vi "Create Landscape.vi"(9 "offset":i32, 10 "Column":i32, 11 "Row":i32) -> ()   [LabVIEW 2016, in "Defenders.lvclass"]
uses:
  Defenders.lvclass
  Terrain.ctl
  Type Defs/Direction Enum.ctl
  SubVIs/Read-Only Globals.vi
  SubVIs/Globals (private).vi
  Landscape Global.vi
  Type Defs/SB Type Defs.lvlib
  Square/Square.lvclass
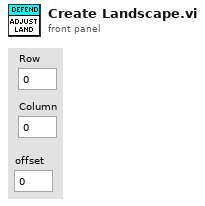
[diagram p1: front panel]
types:
  T1 = typedef "Defenders.lvclass/Terrain.ctl" = enum16{"Wall", "EnemySighted", "EnemyWall", "Mother", "Move", "StagingArea"}
  T2 = typedef "SB Type Defs.lvlib/Direction Enum.ctl" = enum16{"NW", "N", "NE", "E", "SE", "S", "SW", "W"}
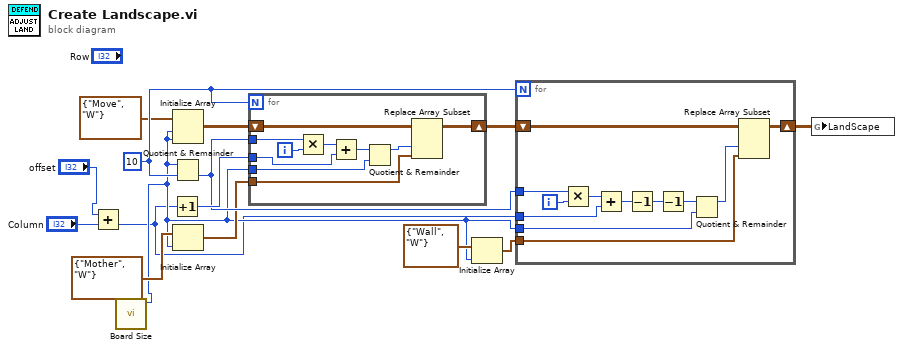
[diagram p0: block diagram]
diagram:
  w14 = 10 ("y")
  n1 = Add(x="offset", y="Column") -> (x+y=w2:i32)
  n2 = call "Board Size.vi"() -> ("Board Size"=w3:i32)  [unwired: 11 in]
  n3 = Increment(x=w2) -> (x+1=w15:i32)
  n4 = Initialize Array(cluster{"Terrain":T1, "Direction":T2} {"Terrain"=enum."Move", "Direction"=enum."W"}, w3, w3) -> (w5:cluster{"Terrain":T1, "Direction":T2}[][])
  n5 = Quotient & Remainder(x=w3, y=w14) -> (floor(x/y)=w13:i32)  [unwired: 1 out]
  n6 = Initialize Array(cluster{"Terrain":T1, "Direction":T2} {"Terrain"=enum."Mother", "Direction"=enum."W"} ("new element/subarray"), w3) -> (w8:cluster{"Terrain":T1, "Direction":T2}[])
  n7 = for {
    N: w14 -> [_]
    tunnel: w8 -> [w24]
    tunnel: w15 -> [w22]
    shift-right: [w23] -> w9
    shift-left: w5 -> [w25]
    tunnel: w13 -> [w20]
    tunnel: w3 -> [w18]
    i -> [w21]
    n8 = Multiply(x=w20, y=w21) -> (x*y=w19:i32)
    n9 = Add(x=w19, y=w22) -> (x+y=w17:i32)
    n10 = Quotient & Remainder(x=w17, y=w18) -> (x-y*floor(x/y)=w16:i32)  [unwired: 1 out]
    n11 = Replace Array Subset(array=w25, new element=w24, index (col)=w16) -> (w23:cluster{"Terrain":T1, "Direction":T2}[][])  [unwired: 1 in]
  }
  n12 = Initialize Array(cluster{"Terrain":T1, "Direction":T2} {"Terrain"=enum."Wall", "Direction"=enum."W"} ("new element/subarray"), w3) -> (w12:cluster{"Terrain":T1, "Direction":T2}[])
  n13 = for {
    N: w14 -> [_]
    tunnel: w12 -> [w36]
    tunnel: w2 -> [w34]
    shift-right: [w35] -> w10
    shift-left: w9 -> [w37]
    tunnel: w13 -> [w32]
    tunnel: w3 -> [w30]
    i -> [w33]
    n14 = Multiply(x=w32, y=w33) -> (x*y=w31:i32)
    n15 = Add(x=w31, y=w34) -> (x+y=w29:i32)
    n16 = Decrement(x=w29) -> (x-1=w27:i32)
    n17 = Decrement(x=w27) -> (x-1=w26:i32)
    n18 = Quotient & Remainder(x=w26, y=w30) -> (x-y*floor(x/y)=w28:i32)  [unwired: 1 out]
    n19 = Replace Array Subset(array=w37, new element=w36, index (col)=w28) -> (w35:cluster{"Terrain":T1, "Direction":T2}[][])  [unwired: 1 in]
  }
  n20 = global write "Landscape Global.vi" "LandScape"(w10) -> ()
